vi "PID.vi"(9 "PID gains in":T4 {"proportional gain (Kc)" format="%.3f"; "integral time (Ti, min)" format="%.3f"; "derivative time (Td, min)" format="%.3f"}, 10 "Ângulo":dbl, 11 "Set-Point":dbl) -> (3 "output":dbl)   [LabVIEW 2015]
uses:
  Desktop/IC/CubeSat/LabView/Control 1.ctl
  Desktop/IC/CubeSat/LabView/Control 2.ctl
  Desktop/IC/CubeSat/LabView/Control 3.ctl
  <vilib>/Simulation/Scripting/Companion Diagram/SimConfigNode/SimParams.ctl
  <vilib>/Simulation/Scripting/Companion Diagram/SimConfigNode/_simSolvers.ctl
  <vilib>/Simulation/Implementation/Shared/SIMSCR Execution Mode.ctl
  <vilib>/Simulation/Param Hierarchy/Typedefs/SIMPH Param Control Actions.ctl
  <vilib>/Simulation/Implementation/Shared/SIM limit type.ctl
  <vilib>/Simulation/Implementation/Shared/NILVSim_ParamChanged.vi
  <vilib>/Simulation/Implementation/Shared/NILVSIM_BeginStep.vi
  <vilib>/Simulation/ContinuousLinear/Implementation/NILVSim Derivative.llb/SIM derivative (scalar).vi
  <vilib>/Simulation/ContinuousLinear/Implementation/NILVSim Integrator new.llb/SIM Integrator distributor (scalar).vi
  <vilib>/Simulation/Nonlinear/Implementation/NILVSim Saturation.llb/SIM Saturation (scalar).vi
  <vilib>/Simulation/ContinuousLinear/Implementation/NILVSim Integrator new.llb/SIM Integrator collector (scalar).vi
  <vilib>/Simulation/Implementation/Shared/NILVSim_Manager.vi
  <vilib>/Utility/error.llb/Clear Errors.vi
  <vilib>/Simulation/Implementation/Shared/NILVSim_FinalizeModel.vi
  <vilib>/Simulation/Implementation/Shared/SIM Unbundle Sim Info.vi
  <vilib>/Simulation/Implementation/Shared/NILVSim_Initialize.vi
  <vilib>/Simulation/Utility/Implementation/NILVSim Get Time and IsAcceptedStep.vi
  <vilib>/Simulation/Implementation/Shared/SIMSH Read Queue.vi
  <vilib>/Simulation/Implementation/Shared/NILVSim_GetModelError.vi
  <vilib>/Simulation/Implementation/Shared/SIM Bundle Sim Info.vi
  <vilib>/Simulation/Scripting/Companion Diagram/SimConfigNode/SimDog.xnode
  <vilib>/Simulation/Implementation/XNodeFramework/SimXNode/SimX.xnode
  <vilib>/Simulation/ContinuousLinear/Implementation/NILVSim Integrator new.llb/SIM Integrator (scalar).vi
  <vilib>/Simulation/Implementation/Shared/NI_SIM_Implementation.lvlib
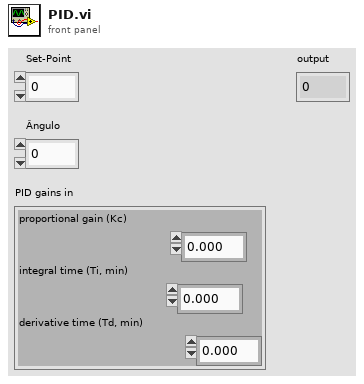
[diagram p1: front panel]
types:
  T1 = typedef "Control 1.ctl" = dbl
  T2 = typedef "Control 2.ctl" = dbl
  T3 = typedef "Control 3.ctl" = dbl
  T4 = cluster{"proportional gain (Kc)":T1, "integral time (Ti, min)":T2, "derivative time (Td, min)":T3}
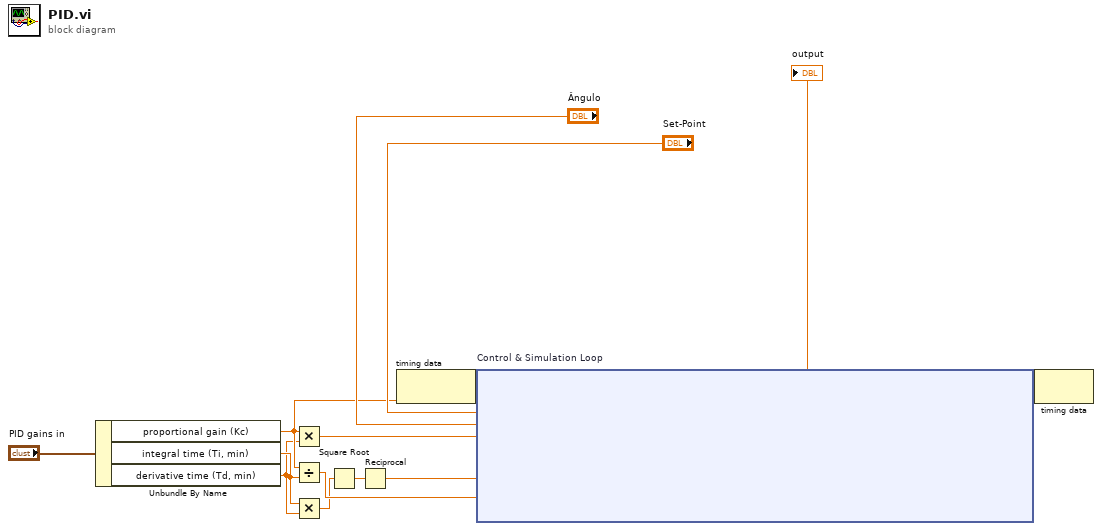
[diagram p0: block diagram]
diagram:
  n1 = Unbundle By Name("PID gains in") -> ("proportional gain (Kc)"=w3:T1, "integral time (Ti, min)"=w7:T2, "derivative time (Td, min)"=w2:T3)
  n2 = Multiply(x=w3, y=w2) -> (x*y=w1:T1)
  n3 = Divide(x=w3, y=w7) -> (x/y=w8:T1)
  n4 = Multiply(x=w7, y=w2) -> (x*y=w6:T2)
  n5 = Square Root(x=w6) -> (sqrt(x)=w5:T2)
  n6 = Reciprocal(x=w5) -> (1/x=w4:T2)
  n7 = node-c288() -> (w14:variant)  [unwired: 1 in]
  n8 = node-c254 "Control & Simulation Loop"(w14, w8, w3, w4, w1, "Set-Point", "Ângulo") -> (w13:variant, →"output":dbl)
  n9 = node-c288(w13) -> ()  [unwired: 1 out]
